vi "Select Camera Dialog.vi"(8 "error in (no error)":errorcluster, 10 "Vendor Name":string[](array[string]), 11 "Camera Name":string[](array[string])) -> (0 "error out":errorcluster, 1 "No camera?":bool caption="OK", 3 "Interface Name":string)   [LabVIEW 2024]
doc: "Okno dialogowe prezentujące wybór wykrytych kamer\nJeśli kamera nie jest obecna, dostarczane są informacje dla użytkownika."
panel:
  out "Camera selected":u16
  in  "OK Button":bool
  in  "Availabe cameras":u16(ring) items=["cam0 USB2.0 FHD UVC WebCam", "cam2 Intel Virtual Camera"]
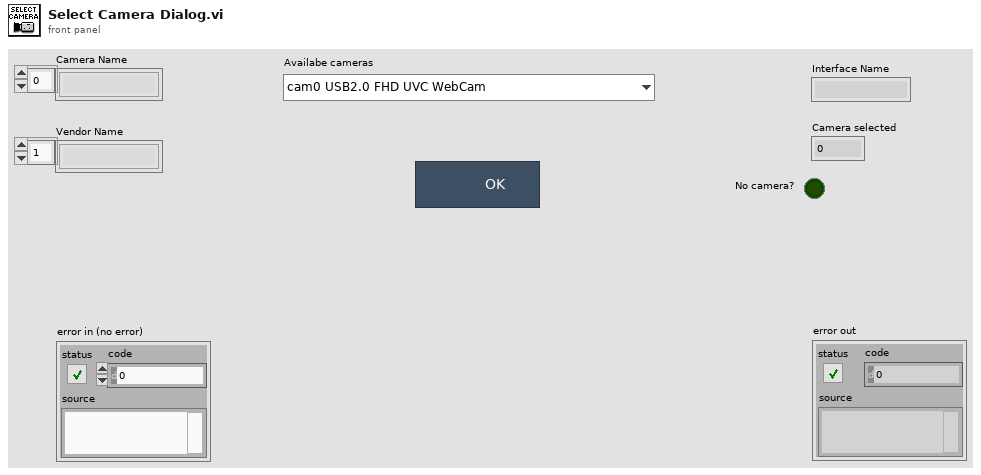
[diagram p1: front panel]
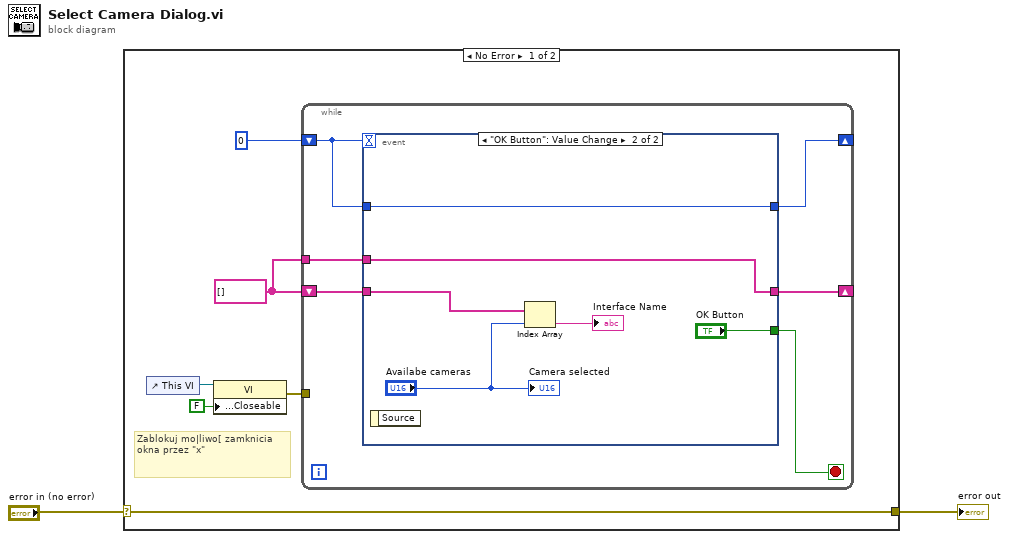
[diagram p0: block diagram]
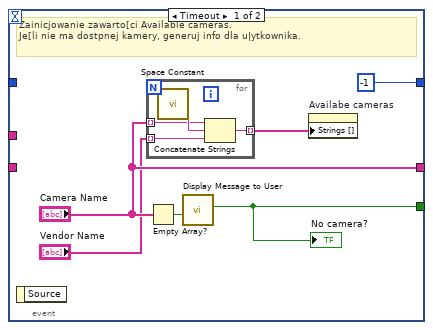
[diagram p2: hidden frame]
diagram:
  n1 = case shown="No Error" "error in (no error)" {
    selector: "error in (no error)" -> [w7 w31]
    tunnel: [w7 w31] -> w1
    frame No Error {
      w6 = string[] [] ("Strings []")
      # "Zablokuj mo|liwo[ zamknicia okna przez \"x\""
      n2 = control-ref of="This VI"() -> (w5:refnum<vi>)
      n3 = property class="VI"(reference=w5, "Front Panel.Closeable"=FALSE ("Front Panel Window:Closeable")) -> (error out=w3:errorcluster)  [unwired: 1 in, 1 out]
      n4 = while {
        shift-right: [w14] -> _
        shift-left: 0 -> [w12]
        shift-right: [w11] -> _
        shift-left: w6 -> [w10]
        tunnel: w6 -> [w9]
        tunnel: w3 -> [_]
        stop <- w13 stop-if-true
        n5 = event shown="[1] \"OK Button\": Value Change" {
          selector: _ -> [_ _]
          dyn-events: _ -> [_ _]
          timeout: w12 -> [_ _]
          tunnel: [-1 w30] -> w14
          tunnel: [w18 "OK Button"] -> w13
          tunnel: w12 -> [_ w30]
          tunnel: ["Camera Name" w26] -> w11
          tunnel: w10 -> [_ w27]
          tunnel: w9 -> [_ w26]
          event Timeout {
            # "Zainicjowanie zawarto[ci Available cameras.\nJe[li nie ma dostpnej kamery, generuj info dla u|ytkownika."
            n6 = event-data() -> ()  [unwired: 1 in, 1 out]
            n7 = for {
              tunnel: "Camera Name" -> [w23] mode=indexing
              tunnel: "Vendor Name" -> [w22] mode=indexing
              tunnel: [w21] -> w15 mode=indexing
              n8 = call <vilib>:"Space Constant.vi"() -> ("String"=w24:string)
              n9 = Concatenate Strings(w23, w24, w22) -> (w21:string)
            }
            n10 = Empty Array?(array="Camera Name") -> (empty?=w19:bool)
            n11 = call "Display Message to User"("Enable"=w19) -> ("OK"=w18:bool)  [unwired: 9 in, 1 out]
            "No camera?" <- w18
            n12 = property on="Availabe cameras" class="Ring (strict)"("Strings []"=w15) -> ()  [unwired: 2 in, 2 out]
          }
          event "OK Button": Value Change {
            n13 = event-data() -> ()  [unwired: 1 in, 1 out]
            n14 = Index Array(array=w27, index="Availabe cameras") -> (element=→"Interface Name":string)
            "Camera selected" <- "Availabe cameras"
          }
        }
      }
    }
    frame Error {
    }
  }
  "error out" <- w1
